vi "Read Version.vi"(11 "ProjectItem in":refnum<class "ProjectItem.lvclass">) -> (1 "Version string":string, 2 "Version":T1, 3 "ProjectItem out":refnum<class "ProjectItem.lvclass">)   [LabVIEW 2019, in "SolutionBuilder.lvlib" / "ProjectItem.lvclass"]
uses:
  ProjectItem.lvclass
  Community/slnbld_BuildSpecVersion.ctl
  ProjectItem.lvclass/ProjectItem.ctl
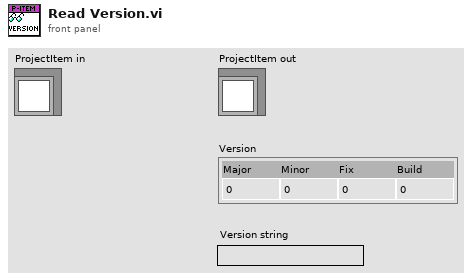
[diagram p1: front panel]
types:
  T1 = typedef "SolutionBuilder.lvlib/ProjectItem.lvclass/slnbld_BuildSpecVersion.ctl" = cluster{"Major":u16, "Minor":u16, "Fix":u16, "Build":u16}
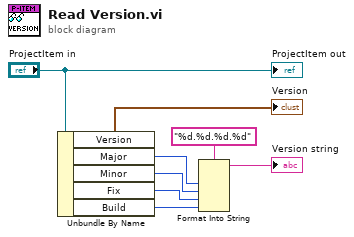
[diagram p0: block diagram]
diagram:
  n1 = Unbundle By Name("ProjectItem in") -> ("Version"=→"Version":T1, "Major"=w3:u16, "Minor"=w4:u16, "Fix"=w5:u16, "Build"=w6:u16)
  n2 = Format Into String(format string="%d.%d.%d.%d", w3, w4, w5, w6) -> (resulting string=→"Version string":string)  [unwired: 2 in, 1 out]
  "ProjectItem out" <- "ProjectItem in"
